vi "仁莫密封检测系统.vi"() -> ()   [LabVIEW 2015]
uses:
  <vilib>/NI/Modbus Library/API/Master/Modbus Master.lvclass
  <vilib>/Utility/file.llb/Read Delimited Spreadsheet (string).vi
  <vilib>/NI/Modbus Library/Transmission Data Unit/RTU/RTU Data Unit.lvclass
  <vilib>/NI/Modbus Library/Master Function Definition/Master Function Definition.lvclass
  <vilib>/NI/Modbus Library/Network Protocol/Network Master/Serial/Serial Master.lvclass
panel:
  out "扫码数据":string
  out "通讯状态":bool
  out "刷新按钮":bool
  out "参数组别":string
  out "测试时间":string
  out "实时压力":string
  out "泄露压力":string
  out "门限压力":string
  out "目标压力":string
  out "测试 NG":string
  out "测试 OK":string
  out "测试结果":string
  out "测试总量":string
  out "实时压力(图)":dbl(graph)
  in  "清除计数":bool
  in  "设备启动":bool
  out "消息框":string
  in  "设备停止":bool
  in  "阻断通讯":bool=TRUE
  out "运行状态":string
  out "失败原因":string
  in  "Exit":bool
  # "仁 莫 密 封 检 测 系 统"
  # "S"
  # "Pa"
  # "Pa"
  # "Pa"
  # "Pa"
  # "pcs"
  # "pcs"
  # "pcs"
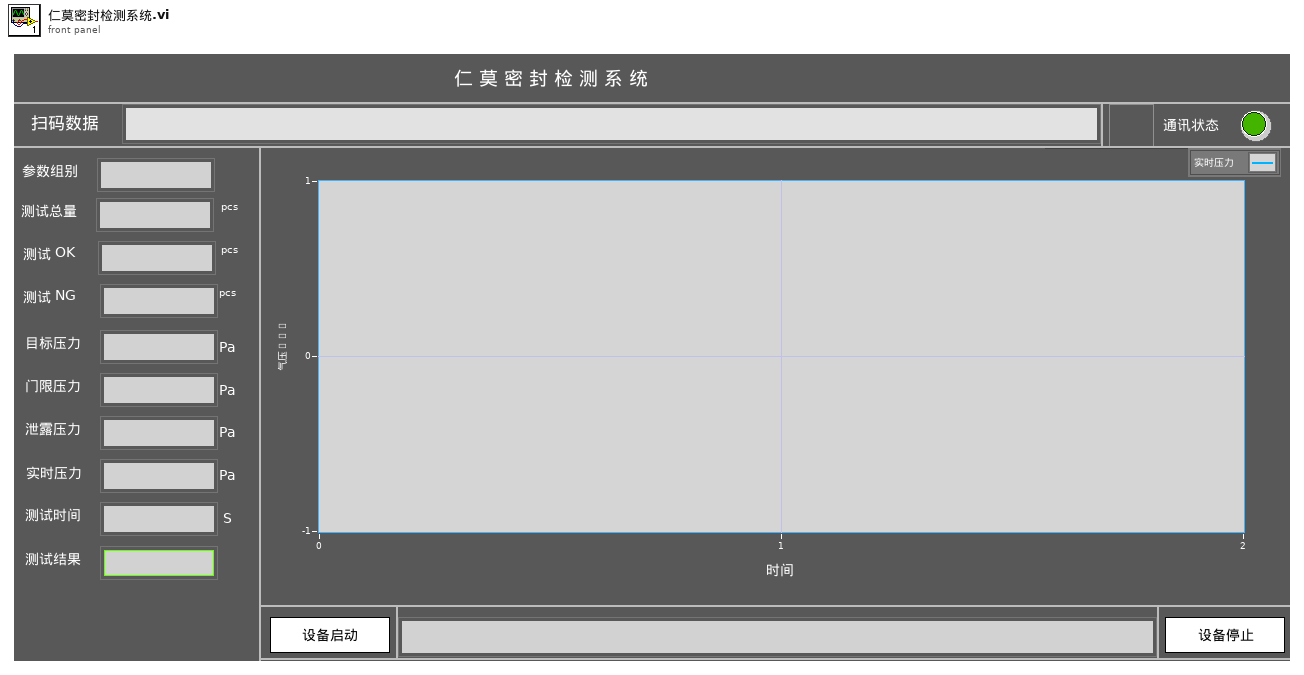
[diagram p1: front panel]
types:
  T1 = cluster{"地址":u16, "数量":u16, "寄存器值":u16[], "产品总数":string}[]
  T2 = enum32{"Invalid", "Standard", "Closed", "Hidden", "Minimized", "Maximized"}
  T3 = enum32{"invalid app kind", "Development System", "Run Time System", "Student Edition", "Embedded LabVIEW", "Evaluation", "Custom"}
  T4 = cluster{"地址":u16, "数量":u16, "寄存器值":u16[], "名称":string}[]
  T5 = cluster{"Core":cluster{"Current VI Reference":refnum<vi>, "Close Panel on Exit?":bool}, "serial master instance":refnum<class "Modbus Master.lvclass">, "进站OK":bool, "连接成功":bool, "正在运行":bool, "用户登录":bool, "A读保持寄存器信息组":cluster{"地址":u16, "数量":u16, "寄存器值":u16[], "名称":string}[], "A写入线圈信息组":cluster{"地址":u16, "布尔":bool, "名称":string}[], "A读多组线圈信息组":cluster{"地址":u16, "数量":u16, "名称":string, "线圈组":bool[]}[]}
  T6 = cluster{"读取信息簇":cluster{"地址":u16, "数量":u16, "寄存器值":u16[], "名称":string}, "值解析":string}[]
  T7 = cluster{"连接成功":bool, "MB_实体":refnum<class "Modbus Master.lvclass">}
  T8 = cluster{"地址":u16, "数量":u16, "名称":string, "线圈组":bool[]}[]
  T9 = cluster{"Current VI Reference":refnum<vi>, "Close Panel on Exit?":bool}
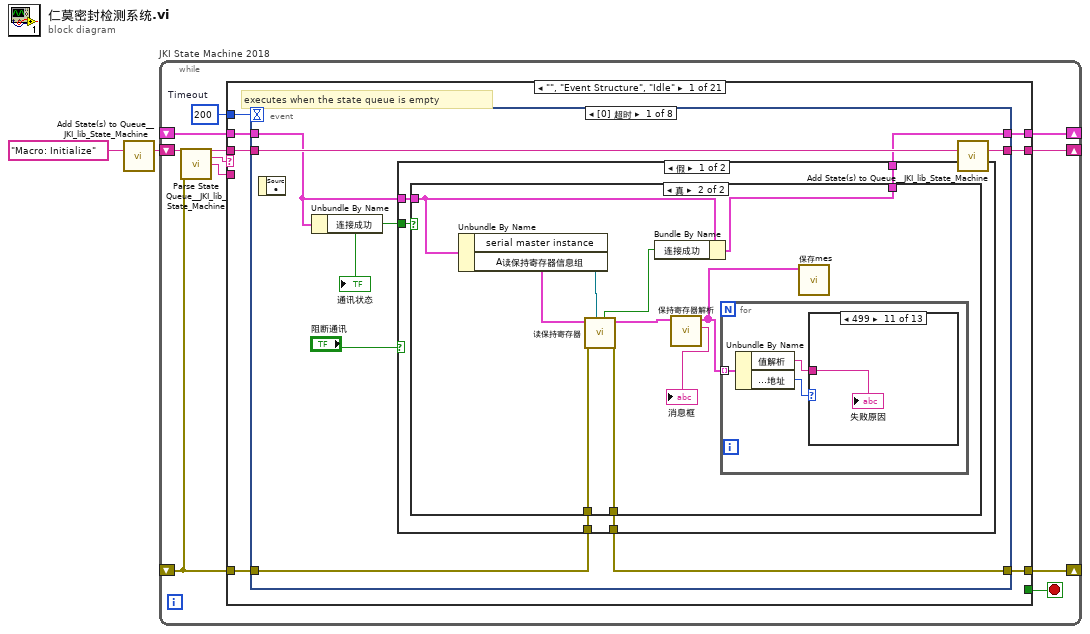
[diagram p0: block diagram]
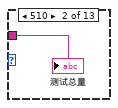
[diagram p4: hidden frame]
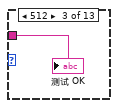
[diagram p5: hidden frame]
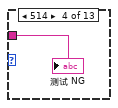
[diagram p6: hidden frame]
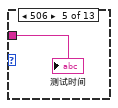
[diagram p7: hidden frame]
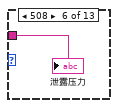
[diagram p8: hidden frame]
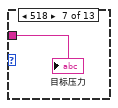
[diagram p9: hidden frame]
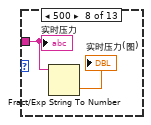
[diagram p10: hidden frame]
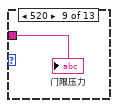
[diagram p11: hidden frame]
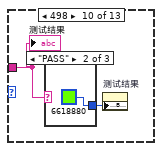
[diagram p12: hidden frame]
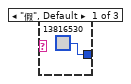
[diagram p13: hidden frame]
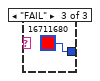
[diagram p14: hidden frame]
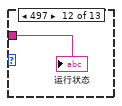
[diagram p15: hidden frame]
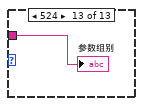
[diagram p16: hidden frame]
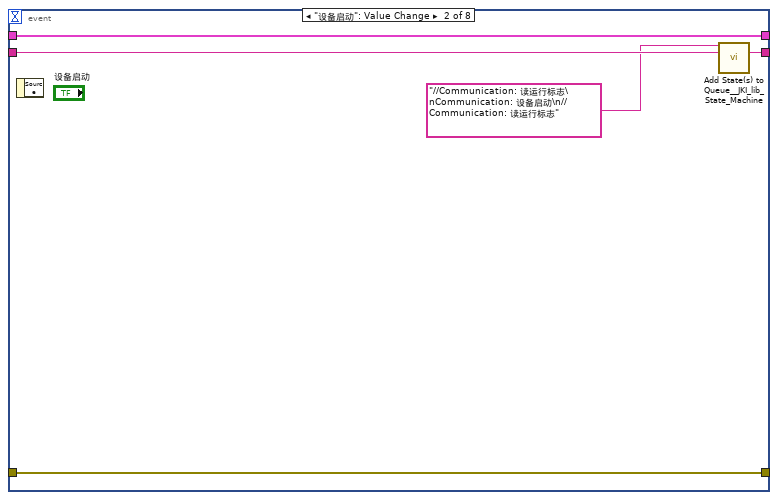
[diagram p18: hidden frame]
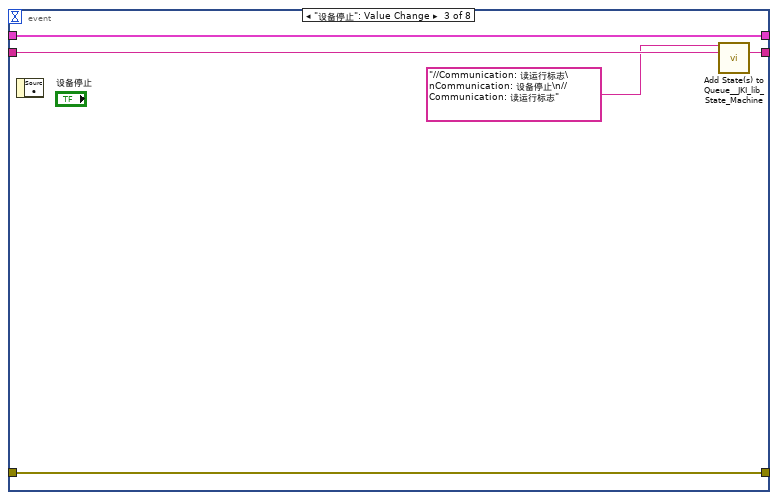
[diagram p19: hidden frame]
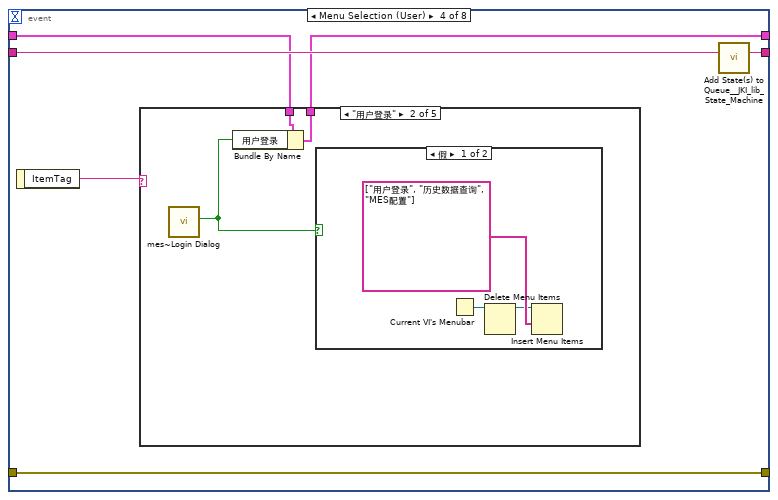
[diagram p20: hidden frame]
diagram:
  n1 = call <vilib>:"Add State(s) to Queue__JKI_lib_State_Machine.vi"("State(s) in (\"\")"="Macro: Initialize") -> ("States Out"=w2:string)  [unwired: 14 in]
  n2 = while "JKI State Machine 2018" {
    shift-right: [w6] -> _
    shift-left: _ -> [w5]
    shift-right: [w9] -> _
    shift-left: _ -> [w3]
    shift-right: [w8] -> _
    shift-left: w2 -> [w10]
    stop <- w7 stop-if-true
    w4 = 200  # Timeout
    n3 = call <vilib>:"Parse State Queue__JKI_lib_State_Machine.vi"("State Queue"=w10, "Error In (no error)"=w3) -> ("Remaining States"=w12:string, "Current State"=w13:string, "Arguments"=w11:string)  [unwired: 11 in]
    n4 = case shown="\"\", \"Event Structure\", \"Idle\"" w13 {
      selector: w13 -> [_ _ w156 _ _ _ _ _ _ _ _ _ _ _ _ _ _ _ _ _ _]
      tunnel: w12 -> [w20 w155 w160 w179 w186 w191 w195 w214 w222 w226 w240 w246 w257 w326 w331 w341 w345 w356 w370 w419 w462]
      tunnel: w11 -> [_ _ _ _ _ _ _ _ _ _ _ w241 w251 _ _ _ _ _ _ _ _]
      tunnel: w5 -> [w18 w152 w158 w172 w183 w189 w192 _ w218 w223 w238 w244 w253 w323 w328 w338 w342 w349 w364 w413 w455]
      tunnel: [w17 w153 w162 w176 errorcluster {"status"=FALSE, "code"=0, "source"=""} ("error out") w188 w193 w211 w219 w224 w237 w242 w254 w324 w329 w339 w343 w350 w367 w416 w459] -> w9
      tunnel: w3 -> [w16 w153 w161 w176 w181 w188 w193 w211 w216 w224 w237 w243 w255 w324 w329 w339 w343 w353 w368 w417 w460]
      tunnel: [w19 w154 w159 w178 w185 w190 w194 w213 w221 w225 w239 w245 w256 w325 w330 w340 w344 w355 w369 w418 w461] -> w8
      tunnel: [_ _ _ _ _ TRUE _ _ _ _ _ _ _ _ _ _ _ _ _ _ _] -> w7
      tunnel: [w15 w152 w158 w177 w183 w189 w192 w212 w218 w223 w238 w244 w253 w323 w328 w338 w342 w347 w362 w411 w456] -> w6
      tunnel: w4 -> [w14 _ _ _ _ _ _ _ _ _ _ _ _ _ _ _ _ _ _ _ _]
      frame "", "Event Structure", "Idle" {
        # "executes when the state queue is empty"
        n5 = event shown="[0] 超时" {
          selector: _ -> [_ _ _ _ _ _ _ _]
          dyn-events: _ -> [_ _ _ _ _ _ _ _]
          timeout: w14 -> [_ _ _ _ _ _ _ _]
          tunnel: w20 -> [w28 w72 w77 w83 w124 w135 w145 w151]
          tunnel: [w27 w71 w76 w82 w123 w134 w144 w150] -> w19
          tunnel: w18 -> [w26 w69 w74 w79 w119 w130 w142 w148]
          tunnel: [w24 w70 w75 w81 w122 w127 w143 w149] -> w17
          tunnel: w16 -> [w25 w70 w75 w81 w122 w128 w143 w149]
          tunnel: [w23 w69 w74 w78 w117 w129 w142 w148] -> w15
          event Timeout {
            n6 = event-data() -> ()  [unwired: 1 in, 1 out]
            n7 = Unbundle By Name(w26) -> ("连接成功"=w21:bool)
            "通讯状态" <- w21
            n8 = case shown="假" "阻断通讯" {
              tunnel: w21 -> [w33 _]
              tunnel: w26 -> [w32 w66]
              tunnel: w25 -> [w31 w67]
              tunnel: [w30 w67] -> w24
              tunnel: [w29 w66] -> w23
              frame False {
                n9 = case shown="真" w33 {
                  tunnel: w32 -> [w35 w43]
                  tunnel: w31 -> [w34 w45]
                  tunnel: [w34 w44] -> w30
                  tunnel: [w35 w37] -> w29
                  frame False {
                  }
                  frame True {
                    n10 = Unbundle By Name(w43) -> ("serial master instance"=w42:refnum<class "Modbus Master.lvclass">, "A读保持寄存器信息组"=w41:T4)
                    n11 = call "读保持寄存器.vi"("MB_实体"=w42, "error in"=w45, "读保持寄存器信息组__输入"=w41) -> ("输出簇"=w44:errorcluster, "读保持寄存器信息组_输出"=w39:T4, "连接成功"=w40:bool)  [unwired: 6 in]
                    n12 = Bundle By Name(cluster=w43, "连接成功"=w40) -> (w37:T5)
                    n13 = call "保持寄存器解析.vi"("A读保持寄存器信息组"=w39) -> ("运行状态"=→"消息框":string, "参数值"=w36:T6)  [unwired: 9 in]
                    n14 = for {
                      tunnel: w36 -> [w47] mode=indexing
                      n15 = Unbundle By Name(w47) -> ("值解析"=w46:string, "读取信息簇.地址"=w48:u16)
                      n16 = case shown="499" w48 {
                        tunnel: w46 -> [_ w49 w50 w51 w52 w53 w54 w56 w57 w59 w63 w64 w65]
                        frame Default {
                        }
                        frame 510 {
                          "测试总量" <- w49
                        }
                        frame 512 {
                          "测试 OK" <- w50
                        }
                        frame 514 {
                          "测试 NG" <- w51
                        }
                        frame 506 {
                          "测试时间" <- w52
                        }
                        frame 508 {
                          "泄露压力" <- w53
                        }
                        frame 518 {
                          "目标压力" <- w54
                        }
                        frame 500 {
                          n17 = Fract/Exp String To Number(string=w56) -> (number=→"实时压力(图)":dbl)  [unwired: 3 in, 1 out]
                          "实时压力" <- w56
                        }
                        frame 520 {
                          "门限压力" <- w57
                        }
                        frame 498 {
                          n18 = case shown="\"PASS\"" w59 {
                            tunnel: [u32 13816530 ("颜色盒") u32 6618880 u32 16711680] -> w58
                            frame "假", Default {
                            }
                            frame "PASS" {
                            }
                            frame "FAIL" {
                            }
                          }
                          n19 = property on="测试结果" class="Str"("Text.BGColor"=w58) -> ()  [unwired: 2 in, 2 out]
                          "测试结果" <- w59
                        }
                        frame 499 {
                          "失败原因" <- w63
                        }
                        frame 497 {
                          "运行状态" <- w64
                        }
                        frame 524 {
                          "参数组别" <- w65
                        }
                      }
                    }
                    n20 = call "保存mes.vi"("参数值"=w36) -> ()  [unwired: 11 in]
                  }
                }
              }
              frame True {
              }
            }
            n21 = call <vilib>:"Add State(s) to Queue__JKI_lib_State_Machine.vi"("State(s) in (\"\")"=w28) -> ("States Out"=w27:string)  [unwired: 14 in]
          }
          event "设备启动": Value Change {
            n22 = event-data() -> ()  [unwired: 1 in, 1 out]
            n23 = call <vilib>:"Add State(s) to Queue__JKI_lib_State_Machine.vi"("State(s) in Front (\"\")"="//Communication: 读运行标志\nCommunication: 设备启动\n//Communication: 读运行标志", "State(s) in (\"\")"=w72) -> ("States Out"=w71:string)  [unwired: 13 in]
          }
          event "设备停止": Value Change {
            n24 = event-data() -> ()  [unwired: 1 in, 1 out]
            n25 = call <vilib>:"Add State(s) to Queue__JKI_lib_State_Machine.vi"("State(s) in Front (\"\")"="//Communication: 读运行标志\nCommunication: 设备停止\n//Communication: 读运行标志", "State(s) in (\"\")"=w77) -> ("States Out"=w76:string)  [unwired: 13 in]
          }
          event Menu Selection (User) {
            n26 = event-data() -> ("ItemTag"=w80:string)  [unwired: 1 in]
            n27 = case shown="\"用户登录\"" w80 {
              tunnel: w79 -> [w84 w87 w95 w106 w108]
              tunnel: [w84 w86 w95 w106 w107] -> w78
              frame "假", Default {
              }
              frame "用户登录" {
                n28 = call "mes~Login Dialog.vi"() -> ("Success?"=w85:bool)  [unwired: 11 in]
                n29 = Bundle By Name(cluster=w87, "用户登录"=w85) -> (w86:T5)
                n30 = case shown="假" w85 {
                  frame False {
                    n31 = Current VI's Menubar() -> (w89:refnum<k9>)
                    n32 = Delete Menu Items(9:w89) -> (3:w88:refnum<k9>)  [unwired: 3 in, 1 out]
                    n33 = Insert Menu Items(7:string[] ["用户登录", "历史数据查询", "MES配置"] ("L10n_item tags 1"), 9:w88) -> ()  [unwired: 4 in, 3 out]
                  }
                  frame True {
                    n34 = Current VI's Menubar() -> (w93:refnum<k9>)
                    n35 = Delete Menu Items(9:w93) -> (0:w91:errorcluster, 3:w92:refnum<k9>)  [unwired: 3 in]
                    n36 = Insert Menu Items(6:w91, 7:string[] ["用户登录", "历史数据查询", "通讯参数设置", "MES配置"] ("L10n_item tags 1"), 9:w92) -> ()  [unwired: 3 in, 3 out]
                  }
                }
              }
              frame "历史数据查询" {
                n37 = stacked-sequence {
                  frame #0 {
                    n38 = call <vilib>:"Check if File or Folder Exists.vi"("path"=path "D:/MES" ("路径")) -> ("file or folder exists?"=w98:bool, "dup path"=w97:path)  [unwired: 8 in, 1 out]
                    n39 = case shown="假" w98 {
                      tunnel: w97 -> [w100 w101]
                      tunnel: [w99 w101] -> _
                      frame False {
                        n40 = Create Folder(path (use dialog)=w100) -> (created path=w99:path)  [unwired: 2 in, 2 out]
                      }
                      frame True {
                      }
                    }
                  }
                  frame #1 {
                    n41 = call <vilib>:"Space Constant.vi"() -> ("String"=w103:string)
                    n42 = Concatenate Strings("explorer" ("字符串"), w103, "D:\\MES" ("字符串")) -> (w105:string)
                    n43 = call <vilib>:"System Exec.vi"("command line"=w105) -> ()  [unwired: 7 in, 4 out]
                  }
                }
              }
              frame "MES配置" {
                n44 = call "mes参数配置.vi"() -> ()  [unwired: 12 in]
              }
              frame "通讯参数设置" {
                n45 = stacked-sequence {
                  tunnel: w108 -> [_ w113 _]
                  tunnel: [_ w110 _] -> w107
                  frame #0 {
                    n46 = local write "阻断通讯"(TRUE ("阻断通讯")) -> ()
                  }
                  frame #1 {
                    n47 = call "通讯参数设置.vi"() -> ("A设备簇"=w114:T7)  [unwired: 5 in]
                    n48 = Unbundle By Name(w114) -> ("MB_实体"=w112:refnum<class "Modbus Master.lvclass">, "连接成功"=w111:bool)
                    n49 = Bundle By Name(cluster=w113, "serial master instance"=w112, "连接成功"=w111) -> (w110:T5)
                  }
                  frame #2 {
                    n50 = local write "阻断通讯"(FALSE ("阻断通讯")) -> ()
                  }
                }
              }
            }
            n51 = call <vilib>:"Add State(s) to Queue__JKI_lib_State_Machine.vi"("State(s) in (\"\")"=w83) -> ("States Out"=w82:string)  [unwired: 14 in]
          }
          event "扫码数据", "刷新按钮": Mouse Down {
            n52 = event-data() -> ()  [unwired: 1 in, 1 out]
            n53 = call "扫码页面.vi"() -> ("Return"=w120:string)  [unwired: 3 in]
            "扫码数据" <- w120
            n54 = global write "Global.vi" "PACK编码"(w120) -> ()
            n55 = call "mes~产品进站.vi"("identification"=w120) -> ("进站成功"=w118:bool)  [unwired: 9 in, 1 out]
            n56 = case shown="真" w118 {
              tunnel: ["产品进站失败，请重新扫码。" "产品进站成功。"] -> w116
              frame False {
              }
              frame True {
              }
            }
            n57 = Bundle By Name(cluster=w119, "进站OK"=w118) -> (w117:T5)
            n58 = local write "消息框"(w116) -> ()
            n59 = call <vilib>:"Add State(s) to Queue__JKI_lib_State_Machine.vi"("State(s) in (\"\")"=w124) -> ("States Out"=w123:string)  [unwired: 14 in]
            "刷新按钮" <- FALSE ("刷新按钮")
          }
          event "清除计数": Value Change {
            n60 = event-data() -> ()  [unwired: 1 in, 1 out]
            n61 = local write "清除计数"(FALSE) -> ()
            n62 = Unbundle By Name(w130) -> ("serial master instance"=w131:refnum<class "Modbus Master.lvclass">)
            n63 = disable-structure shown="禁用" {
              disable-tunnel: [w140 _] -> w132
              disable-tunnel: w131 -> [w139 _]
              disable-tunnel: w128 -> [w137 _]
              disable-tunnel: [w136 _] -> w127
              frame Disabled {
                n64 = call "写保持寄存器.vi"("MB_实体"=w139, "error in"=w137, "读保持寄存器信息组__输入"=T1 [{"地址"=510, "数量"=2, "寄存器值"=[0, 0], "产品总数"="产品总数"}, {"地址"=512, "数量"=2, "寄存器值"=[0, 0], "产品总数"="合格数量"}, {"地址"=514, "数量"=2, "寄存器值"=[0, 0], "产品总数"="泄露数量"}]) -> ("输出簇"=w136:errorcluster, "连接成功"=w140:bool)  [unwired: 7 in]
              }
              frame Enabled {
              }
            }
            n65 = Bundle By Name(cluster=w130, "连接成功"=w132) -> (w129:T5)
            n66 = call <vilib>:"Add State(s) to Queue__JKI_lib_State_Machine.vi"("State(s) in (\"\")"=w135) -> ("States Out"=w134:string)  [unwired: 14 in]
          }
          event "Exit": Value Change {
            # "Exit Button Value Change (pressed) Event\n(this executes Macro: Exit to terminate the VI)"
            n67 = event-data() -> ()  [unwired: 1 in, 1 out]
            n68 = call <vilib>:"Add State(s) to Queue__JKI_lib_State_Machine.vi"("State(s) in Front (\"\")"="Macro: Exit", "State(s) in (\"\")"=w145) -> ("States Out"=w144:string)  [unwired: 13 in]
          }
          event Panel Close? {
            # "Discard the event because we'll close the front panel ourselves in Macro: Exit"
            # "Close Panel button (pressed) Event\n(this executes Macro: Exit to terminate the VI)"
            n69 = event-data() -> ()  [unwired: 1 in, 1 out]
            n70 = event-data("Discard?"=TRUE) -> ()  [unwired: 1 in, 1 out]
            n71 = call <vilib>:"Add State(s) to Queue__JKI_lib_State_Machine.vi"("State(s) in Front (\"\")"="Macro: Exit", "State(s) in (\"\")"=w151) -> ("States Out"=w150:string)  [unwired: 13 in]
          }
        }
      }
      frame "---------- Core ----------" {
        # "Do not put any code in this frame.\n(it is a separator no-op)"
        n72 = call <vilib>:"Add State(s) to Queue__JKI_lib_State_Machine.vi"("State(s) in (\"\")"=w155) -> ("States Out"=w154:string)  [unwired: 14 in]
      }
      frame Default {
        w165 = 42 items=["No error", "Argument error", "Memory is full", "Out of zone", "End of file", "File already open", "Generic file I/O error", "File not found", "File permission error", "Disk is full", "Duplicate path", "Too many files open", "System feature not enabled", "Resource file not found", "Cannot add resource", "Resource not found", "Image not found", "Image memory error", "Pen does not exist", "Config type invalid", "Config token not found", "Config parse error", "Config memory error", "Bad external code format", "Bad external code offset", "External code not present", "Null window", "Destroy window error", "Null menu", "Print aborted", "Bad print record", "Print driver error", "Windows error during printing", "Memory error during printing", "Print dialog error", "Generic print error", "Invalid device refnum", "Device not found", "Device parameter error", "Device unit error", "Cannot open device", "Device call aborted", "Generic error", "Cancelled by user", "Object ID too low", "Object ID too high", "Object not in heap", "Unknown heap", "Unknown object (invalid DefProc)", "Unknown object (DefProc not in table)", "Message out of range", "Invalid (null) method", "Unknown message", "Manager call not supported", "Bad address", "Network operation in progress", "Network operation timed out", "Connection is busy", "Network attribute not supported", "Network error", "Address in use", "System out of memory", "Connection aborted", "Connection refused", "Not connected", "Already connected", "Connection closed", "Initialization error (interapplication manager)", "Bad occurrence", "Wait on unbound occurrence handler", "Occurrence queue overflow", "Datalog type conflict", "Unused", "Unrecognized type (interapplication manager)", "Memory corrupt", "Failed to make temporary DLL", "Old CIN version", "Drag socket not found", "Failed to load drop-object", "Failed to register OLE object", "Failed to release OLE object", "Format specifier type mismatch", "Unknown format specifier", "Too few format specifiers", "Too many format specifiers", "Scan failed", "Newer CIN version", "Error converting to variant", "Runtime menu error", "Password tampered", "Variant attribute not found", "Incompatible variant data type", "Event data is not available", "Event Store is not present", "Occurrence is not found", "Event Queue is not created", "Event info is not available", "Refnum passed is NULL", "Error retrieving Class GUID", "Error retrieving CoClass GUID", "Error retrieving TypeLib GUID.", "Bad built application magic bytes.", "Specific driver is different from the specific driver associated with the Logical Name.", "There is no session opened to the class driver.", "Max Error", "MAX - Error with config objects", "MAX - Error loading configuration", "MAX - Group not supported"]
        # "Current State"
        # "Do not delete, rename, or modify this frame.\n(this is used to capture unhandled states and typos)"
        # "Handle mistyped state name (developer tool)"
        n73 = Format Into String(format string="Software Exception: Unhandled State \"%s\"." ("message"), error in=w161, w156) -> (resulting string=w164:string, error out=w163:errorcluster)  [unwired: 1 in]
        n74 = call <vilib>:"Error Cluster From Error Code.vi"("show call chain? (False)"=TRUE, "error in (no error)"=w163, "error message (\"\")"=w164, "error code (0)"=w165) -> ("error out"=w162:errorcluster)  [unwired: 5 in]
        n75 = call <vilib>:"Add State(s) to Queue__JKI_lib_State_Machine.vi"("State(s) in (\"\")"=w160) -> ("States Out"=w159:string)  [unwired: 14 in]
      }
      frame "Initialize Core Data" {
        # "Do not delete, rename, or modify this frame.\n(this is used to determine panel behavior on exit)"
        # "originally closed?"
        # "exe?"
        # "If panel starts closed or is an EXE, then close it when we exit"
        n76 = property class="VI"() -> ("FP.State"=w169:T2)  [unwired: 2 in, 2 out]
        n77 = property class="App"() -> ("App.Kind"=w175:T3)  [unwired: 2 in, 2 out]
        n78 = control-ref of="Current VI Reference"() -> (w170:refnum<vi>)
        n79 = Equal?(x=w169, y=T2."Closed" ("Front Panel Window:State")) -> (x = y?=w167:bool)
        n80 = Equal?(x=w175, y=T3."Run Time System" ("Application:Kind")) -> (x = y?=w173:bool)
        n81 = Or(x=w167, y=w173) -> (x .or. y?=w171:bool)
        n82 = Bundle By Name(cluster=w172, "Core.Current VI Reference"=w170, "Core.Close Panel on Exit?"=w171) -> (w177:T5)
        n83 = call <vilib>:"Add State(s) to Queue__JKI_lib_State_Machine.vi"("State(s) in (\"\")"=w179) -> ("States Out"=w178:string)  [unwired: 14 in]
      }
      frame "Error Handler" {
        # "Handle any errors here.\nYou can also output any states to clean-up after errors occur"
        # "Clear error"
        n84 = Unbundle By Name(w181) -> ("source"=w180:string)
        n85 = One Button Dialog(message=w180) -> ()  [unwired: 1 in, 1 out]
        n86 = call <vilib>:"Add State(s) to Queue__JKI_lib_State_Machine.vi"("State(s) in Front (\"\")"="/* Post Error States", "State(s) in (\"\")"=w186) -> ("States Out"=w185:string)  [unwired: 13 in]
      }
      frame "Exit" {
        # "Do not put any code in this frame.\n(No errors that occur here will be handled.)"
        n87 = call <vilib>:"Add State(s) to Queue__JKI_lib_State_Machine.vi"("State(s) in (\"\")"=w191) -> ("States Out"=w190:string)  [unwired: 14 in]
      }
      frame "---------- Data ----------" {
        # "Do not put any code in this frame.\n(It is a separator no-op. You can make a copy of this frame to create a new Data frame)"
        n88 = call <vilib>:"Add State(s) to Queue__JKI_lib_State_Machine.vi"("State(s) in (\"\")"=w195) -> ("States Out"=w194:string)  [unwired: 14 in]
      }
      frame "Data: Initialize" {
        w196 = FALSE  # 进站OK
        w203 = FALSE  # 用户登录
        w204 = FALSE  # 正在运行
        w205 = T4 [{"地址"=510, "数量"=2, "寄存器值"=[0, 0], "名称"="产品总数"}, {"地址"=512, "数量"=2, "寄存器值"=[0, 0], "名称"="合格数量"}, {"地址"=514, "数量"=2, "寄存器值"=[0, 0], "名称"="泄露数量"}, {"地址"=506, "数量"=2, "寄存器值"=[0, 0], "名称"="1测试时间"}, {"地址"=508, "数量"=2, "寄存器值"=[0, 0], "名称"="1测试泄漏"}, {"地址"=518, "数量"=2, "寄存器值"=[0, 0], "名称"="1#目标压力"}, {"地址"=498, "数量"=1, "寄存器值"=[0, 0], "名称"="1#测试结果"}, {"地址"=500, "数量"=2, "寄存器值"=[0, 0], "名称"="实时压力"}, {"地址"=520, "数量"=2, "寄存器值"=[], "名称"="门限压力"}, {"地址"=499, "数量"=1, "寄存器值"=[], "名称"="失败原因"}, {"地址"=497, "数量"=1, "寄存器值"=[], "名称"="运行状态"}, {"地址"=524, "数量"=2, "寄存器值"=[], "名称"="参数组别"}]  # A读保持寄存器信息组
        w206 = T8 [{"地址"=507, "数量"=1, "名称"="1测试结束标志", "线圈组"=[FALSE, TRUE]}]  # A读多组线圈信息组
        w207 = cluster{"地址":u16, "布尔":bool, "名称":string}[] [{"地址"=50, "布尔"=FALSE, "名称"="启动"}, {"地址"=51, "布尔"=FALSE, "名称"="停止"}]  # A写入线圈信息组
        w208 = FALSE  # 连接成功
        w209 = refnum<class "Modbus Master.lvclass"> refnum  # serial master instance
        w210 = T9 {"Current VI Reference"=refnum, "Close Panel on Exit?"=FALSE}  # Core
        # "Data names and types of shift register data are defined by this bundle."
        # "Initialize the shift-register data, here.\n(data names are defined by what you wire into the bundle function)"
        n89 = call <vilib>:"Application Directory.vi"() -> ("Application Directory"=w201:path)
        n90 = Build Path(base path=w201, name or relative path=path "data/mes.cfg") -> (appended path=w202:path)
        n91 = call-poly <vilib>:"Read Delimited Spreadsheet.vi"("file path (dialog if empty)"=w202, "delimiter (\\t)"="::" ("delimiter (\\t)")) -> ("all rows"=w197:string[][])  [unwired: 8 in, 5 out]
        n92 = call "mes初始化.vi"("mes"=w197) -> ()  [unwired: 11 in]
        n93 = global write "Global.vi" "运行状态时间点"(dbl[] [0.0, 0.0, 0.0, 0.0, 0.0, 0.0, 0.0, 0.0, 0.0] ("运行状态时间点")) -> ()
        n94 = Bundle("Core"=w210, "serial master instance"=w209, "进站OK"=w196, "连接成功"=w208, "正在运行"=w204, "用户登录"=w203, "A读保持寄存器信息组"=w205, "A写入线圈信息组"=w207, "A读多组线圈信息组"=w206) -> (w212:T5)  [unwired: 1 in]
        n95 = call <vilib>:"Add State(s) to Queue__JKI_lib_State_Machine.vi"("State(s) in (\"\")"=w214) -> ("States Out"=w213:string)  [unwired: 14 in]
      }
      frame "Data: Cleanup" {
        # "Cleanup any data and references, here.\n(this is called automatically, by the Macro: Exit)"
        n96 = Unbundle By Name(w218) -> ("Core.Current VI Reference"=w220:refnum<vi>, "serial master instance"=w217:refnum<class "Modbus Master.lvclass">)
        n97 = call-dynamic "Shutdown.vi"("error in"=w216, "Modbus master in"=w217) -> ("error out"=w215:errorcluster)  [unwired: 9 in]
        n98 = Close Reference(reference=w220, error in (no error)=w215) -> (error out=w219:errorcluster)
        n99 = call <vilib>:"Add State(s) to Queue__JKI_lib_State_Machine.vi"("State(s) in (\"\")"=w222) -> ("States Out"=w221:string)  [unwired: 14 in]
      }
      frame "---------- UI ----------" {
        # "Do not put any code in this frame.\n(It is a separator no-op. You can make a copy of this frame to create a new UI frame)"
        n100 = call <vilib>:"Add State(s) to Queue__JKI_lib_State_Machine.vi"("State(s) in (\"\")"=w226) -> ("States Out"=w225:string)  [unwired: 14 in]
      }
      frame "UI: Initialize" {
        w232 = ""
        # "Initialize the User Interface, here.\n(this is called automatically, by the Macro: Init)"
        n101 = call "读取配置文件.vi"("配置"="程序名") -> ("error out"=w231:errorcluster, "路径"=w230:string)  [unwired: 9 in]
        n102 = property class="VI"(error in=w231, "Front Panel.Title"=w230) -> (error out=w228:errorcluster)  [unwired: 1 in, 1 out]
        n103 = Current VI's Menubar() -> (w236:refnum<k9>)
        n104 = Delete Menu Items(6:w228, 9:w236) -> (0:w235:errorcluster, 3:w234:refnum<k9>)  [unwired: 2 in]
        n105 = local write "扫码数据"(w232) -> ()
        n106 = global write "Global.vi" "PACK编码"(w232) -> ()
        n107 = Insert Menu Items(6:w235, 7:string[] ["用户登录", "历史数据查询", "MES配置"] ("L10n_item tags 1"), 9:w234) -> ()  [unwired: 3 in, 3 out]
        n108 = property on="测试结果" class="Str"("Text.BGColor"=u32 13816530 ("颜色盒")) -> ()  [unwired: 2 in, 2 out]
        n109 = call <vilib>:"Add State(s) to Queue__JKI_lib_State_Machine.vi"("State(s) in (\"\")"=w240) -> ("States Out"=w239:string)  [unwired: 14 in]
      }
      frame "UI: Cursor Set" {
        # "Argument"
        # "Set and Unset Cursor Busy.\n(Usage: \"UI: Cursor Set >> Busy|Idle\")"
        n110 = case shown="\"Idle\", 默认" w241 {
          tunnel: w243 -> [w248 w250]
          tunnel: [w247 w249] -> w242
          frame "Idle", Default {
            n111 = call <vilib>:"Unset Busy.vi"("error in (no error)"=w248) -> ("error out"=w247:errorcluster)  [unwired: 10 in]
          }
          frame "Busy" {
            n112 = call <vilib>:"Set Busy.vi"("error in (no error)"=w250) -> ("error out"=w249:errorcluster)  [unwired: 9 in, 1 out]
          }
        }
        n113 = call <vilib>:"Add State(s) to Queue__JKI_lib_State_Machine.vi"("State(s) in (\"\")"=w246) -> ("States Out"=w245:string)  [unwired: 14 in]
      }
      frame "UI: Front Panel State" {
        # "Argument"
        # "Set Front Panel Open or Closed\n(Usage: \"UI: Front Panel State >> Open|Close\")"
        n114 = Unbundle By Name(w253) -> ("Core.Current VI Reference"=w252:refnum<vi>)
        n115 = case shown="\"Maximize\", \"Maximized\"" w251 {
          tunnel: w255 -> [w263 w278 w289 w302 w315]
          tunnel: [w265 w279 w291 w304 w317] -> w254
          tunnel: w252 -> [w264 w276 w290 w303 w316]
          frame "Open", "Standard", Default {
            w258 = T2."Standard" ("State")
            n116 = property class="VI"(reference=w264, error in=w263) -> (reference out=w261:refnum<vi>, error out=w262:errorcluster, "FP.State"=w260:T2)
            n117 = Not Equal?(x=w260, y=w258) -> (x != y?=w259:bool)
            n118 = case shown="真" w259 {
              tunnel: [w269 w271] -> w265
              tunnel: w262 -> [w268 w271]
              tunnel: w261 -> [w267 _]
              tunnel: w258 -> [w266 _]
              frame True {
                n119 = invoke class="VI" method="FP.Open"(reference=w267, error in=w268, "Activate"=TRUE, "State"=w266) -> (error out=w269:errorcluster)  [unwired: 1 in, 4 out]
              }
              frame False {
              }
            }
          }
          frame "Close", "Closed" {
            n120 = property class="VI"(reference=w276, error in=w278) -> (reference out=w275:refnum<vi>, error out=w277:errorcluster, "FP.State"=w273:T2)
            n121 = Not Equal?(x=w273, y=T2."Closed" ("Front Panel Window:State")) -> (x != y?=w272:bool)
            n122 = case shown="真" w272 {
              tunnel: [w280 w283] -> w279
              tunnel: w277 -> [w280 w282]
              tunnel: w275 -> [_ w281]
              frame False {
              }
              frame True {
                n123 = invoke class="VI" method="FP.Close"(reference=w281, error in=w282) -> (error out=w283:errorcluster)  [unwired: 1 in, 2 out]
              }
            }
          }
          frame "Hidden", "Hide" {
            w284 = T2."Hidden" ("State")
            n124 = property class="VI"(reference=w290, error in=w289) -> (reference out=w287:refnum<vi>, error out=w288:errorcluster, "FP.State"=w286:T2)
            n125 = Not Equal?(x=w286, y=w284) -> (x != y?=w285:bool)
            n126 = case shown="真" w285 {
              tunnel: [w295 w296] -> w291
              tunnel: w288 -> [w294 w296]
              tunnel: w287 -> [w293 _]
              tunnel: w284 -> [w292 _]
              frame True {
                n127 = invoke class="VI" method="FP.Open"(reference=w293, error in=w294, "State"=w292) -> (error out=w295:errorcluster)  [unwired: 2 in, 4 out]
              }
              frame False {
              }
            }
          }
          frame "Minimize", "Minimized" {
            w297 = T2."Minimized" ("State")
            n128 = property class="VI"(reference=w303, error in=w302) -> (reference out=w300:refnum<vi>, error out=w301:errorcluster, "FP.State"=w299:T2)
            n129 = Not Equal?(x=w299, y=w297) -> (x != y?=w298:bool)
            n130 = case shown="真" w298 {
              tunnel: [w308 w309] -> w304
              tunnel: w301 -> [w307 w309]
              tunnel: w300 -> [w306 _]
              tunnel: w297 -> [w305 _]
              frame True {
                n131 = invoke class="VI" method="FP.Open"(reference=w306, error in=w307, "State"=w305) -> (error out=w308:errorcluster)  [unwired: 2 in, 4 out]
              }
              frame False {
              }
            }
          }
          frame "Maximize", "Maximized" {
            w310 = T2."Maximized" ("State")
            n132 = property class="VI"(reference=w316, error in=w315) -> (reference out=w313:refnum<vi>, error out=w314:errorcluster, "FP.State"=w312:T2)
            n133 = Not Equal?(x=w312, y=w310) -> (x != y?=w311:bool)
            n134 = case shown="真" w311 {
              tunnel: [w321 w322] -> w317
              tunnel: w314 -> [w320 w322]
              tunnel: w313 -> [w319 _]
              tunnel: w310 -> [w318 _]
              frame True {
                n135 = invoke class="VI" method="FP.Open"(reference=w319, error in=w320, "State"=w318) -> (error out=w321:errorcluster)  [unwired: 2 in, 4 out]
              }
              frame False {
              }
            }
          }
        }
        n136 = call <vilib>:"Add State(s) to Queue__JKI_lib_State_Machine.vi"("State(s) in (\"\")"=w257) -> ("States Out"=w256:string)  [unwired: 14 in]
      }
      frame "---------- Macro ----------" {
        # "Do not put any code in this frame.\n(It is a separator no-op. You can make a copy of this frame to create a new Macro frame)"
        n137 = call <vilib>:"Add State(s) to Queue__JKI_lib_State_Machine.vi"("State(s) in (\"\")"=w326) -> ("States Out"=w325:string)  [unwired: 14 in]
      }
      frame "Macro: Initialize" {
        w327 = "Data: Initialize\nInitialize Core Data\nUI: Initialize\nUI: Front Panel State >> Maximize\nCommunication: Open Serial\nCommunication: 读运行标志"  # Data: Initialize Initialize Core Data UI: Initialize UI: Front Panel State >> Maximize Communication: Open Serial Communication: 读运行标志
        # "Initialization Macro\n(This is called once, when the VI starts)"
        n138 = call <vilib>:"Add State(s) to Queue__JKI_lib_State_Machine.vi"("State(s) in Front (\"\")"=w327, "State(s) in (\"\")"=w331) -> ("States Out"=w330:string)  [unwired: 13 in]
      }
      frame "Macro: Exit" {
        # "Exit Macro\n(This is called once, when the VI exits)"
        n139 = Unbundle By Name(w338) -> ("Core.Close Panel on Exit?"=w337:bool)
        n140 = Select(t="UI: Front Panel State >> Close", s=w337, f="") -> (s? t:f=w334:string)
        n141 = call <vilib>:"Add State(s) to Queue__JKI_lib_State_Machine.vi"("State(s) in (\"\")"=w334, "State(s) at Back (\"\")"="Data: Cleanup\nExit") -> ("States Out"=w332:string)  [unwired: 13 in]
        n142 = call <vilib>:"Add State(s) to Queue__JKI_lib_State_Machine.vi"("State(s) in Front (\"\")"=w332, "State(s) in (\"\")"=w341) -> ("States Out"=w340:string)  [unwired: 13 in]
      }
      frame "---------- Communication ----------" {
        # "Template Separator\n(You can make a copy of, or modify, this frame)"
        n143 = call <vilib>:"Add State(s) to Queue__JKI_lib_State_Machine.vi"("State(s) in (\"\")"=w345) -> ("States Out"=w344:string)  [unwired: 14 in]
      }
      frame "Communication: Open Serial" {
        # "Your code here.\n(You can make a copy of, or modify, this frame)"
        n144 = call "读取配置文件.vi"("error in"=w353, "配置"="串口号") -> ("error out"=w352:errorcluster, "路径"=w351:string)  [unwired: 8 in]
        n145 = call "开机连接.vi"("error in"=w352, "串口号"=w351) -> ("error out"=w350:errorcluster, "连接成功"=w346:bool, "serial master instance"=w348:refnum<class "Modbus Master.lvclass">)  [unwired: 7 in]
        n146 = Bundle By Name(cluster=w349, "serial master instance"=w348, "连接成功"=w346) -> (w347:T5)
        n147 = call <vilib>:"Add State(s) to Queue__JKI_lib_State_Machine.vi"("State(s) in (\"\")"=w356) -> ("States Out"=w355:string)  [unwired: 14 in]
      }
      frame "Communication: 设备启动" {
        # "Your code here.\n(You can make a copy of, or modify, this frame)"
        n148 = Unbundle By Name(w364) -> ("serial master instance"=w365:refnum<class "Modbus Master.lvclass">, "连接成功"=w366:bool, "用户登录"=w358:bool, "进站OK"=w357:bool)
        n149 = And(x=w358, y=w357) -> (x .and. y?=w359:bool)
        n150 = case shown="假" w359 {
          tunnel: w368 -> [w373 w385]
          tunnel: [w373 w384] -> w367
          tunnel: w366 -> [w374 w383]
          tunnel: w365 -> [_ w382]
          tunnel: [w374 w381] -> w363
          tunnel: FALSE ("正在运行") -> [w375 w380]
          tunnel: [w375 w379] -> w361
          tunnel: w358 -> [w372 _]
          tunnel: w357 -> [w371 _]
          frame False {
            n151 = case shown="真" w372 {
              tunnel: w371 -> [_ w377]
              frame False {
                n152 = One Button Dialog(message="用户未登录" ("消息")) -> ()  [unwired: 1 in, 1 out]
              }
              frame True {
                n153 = case shown="真" w377 {
                  frame False {
                  }
                  frame True {
                    n154 = One Button Dialog(message="进站失败。" ("消息")) -> ()  [unwired: 1 in, 1 out]
                  }
                }
              }
            }
          }
          frame True {
            n155 = case shown="假" w380 {
              selector: w380 -> [_ w405]
              tunnel: w385 -> [w391 w406]
              tunnel: [w390 w406] -> w384
              tunnel: w383 -> [w389 w407]
              tunnel: w382 -> [w388 _]
              tunnel: [w387 w407] -> w381
              tunnel: [w386 w405] -> w379
              frame False {
                n156 = case shown="真" w389 {
                  tunnel: w391 -> [w392 w397]
                  tunnel: [w392 w396] -> w390
                  tunnel: w388 -> [_ w395]
                  tunnel: [_ w394] -> w387
                  tunnel: [_ TRUE] -> w386
                  frame False {
                  }
                  frame True {
                    n157 = stacked-sequence {
                      tunnel: w397 -> [_ w403 _]
                      tunnel: [_ w402 _] -> w396
                      tunnel: w395 -> [_ w401 _]
                      tunnel: [_ w400 _] -> w394
                      frame #0 {
                        n158 = local write "阻断通讯"(TRUE ("阻断通讯")) -> ()
                      }
                      frame #1 {
                        w399 = cluster{"地址":u16, "布尔":bool, "名称":string}[] [{"地址"=50, "布尔"=TRUE, "名称"="启动"}, {"地址"=51, "布尔"=FALSE, "名称"="停止"}]  # A写入线圈信息组
                        n159 = call "写入单个线圈.vi"("error in"=w403, "写入线圈信息组"=w399, "MB_实体"=w401) -> ("输出簇"=w402:errorcluster, "连接成功"=w400:bool)  [unwired: 7 in]
                      }
                      frame #2 {
                        n160 = local write "阻断通讯"(FALSE ("阻断通讯")) -> ()
                      }
                    }
                  }
                }
              }
              frame True {
              }
            }
          }
        }
        n161 = Bundle By Name(cluster=w364, "正在运行"=w361, "连接成功"=w363) -> (w362:T5)
        n162 = call <vilib>:"Add State(s) to Queue__JKI_lib_State_Machine.vi"("State(s) in (\"\")"=w370) -> ("States Out"=w369:string)  [unwired: 14 in]
      }
      frame "Communication: 设备停止" {
        # "Your code here.\n(You can make a copy of, or modify, this frame)"
        n163 = Unbundle By Name(w413) -> ("serial master instance"=w414:refnum<class "Modbus Master.lvclass">, "连接成功"=w415:bool, "用户登录"=w409:bool)
        n164 = case shown="真" w409 {
          tunnel: w417 -> [w422 w430]
          tunnel: [w422 w429] -> w416
          tunnel: w415 -> [w420 w428]
          tunnel: w414 -> [_ w427]
          tunnel: [w420 w426] -> w412
          tunnel: TRUE ("正在运行") -> [w421 w425]
          tunnel: [w421 w424] -> w410
          frame False {
            n165 = One Button Dialog(message="用户未登录" ("消息")) -> ()  [unwired: 1 in, 1 out]
          }
          frame True {
            n166 = case shown="真" w425 {
              selector: w425 -> [w431 _]
              tunnel: w430 -> [w432 w439]
              tunnel: [w432 w438] -> w429
              tunnel: w428 -> [w433 w437]
              tunnel: w427 -> [_ w436]
              tunnel: [w433 w435] -> w426
              tunnel: [w431 w434] -> w424
              frame False {
              }
              frame True {
                n167 = case shown="真" w437 {
                  tunnel: w439 -> [w441 w446]
                  tunnel: [w441 w445] -> w438
                  tunnel: w436 -> [_ w444]
                  tunnel: [_ w443] -> w435
                  tunnel: [FALSE FALSE] -> w434
                  frame False {
                  }
                  frame True {
                    n168 = stacked-sequence {
                      tunnel: w446 -> [_ w452 _]
                      tunnel: [_ w451 _] -> w445
                      tunnel: w444 -> [_ w450 _]
                      tunnel: [_ w449 _] -> w443
                      frame #0 {
                        n169 = local write "阻断通讯"(TRUE ("阻断通讯")) -> ()
                      }
                      frame #1 {
                        w448 = cluster{"地址":u16, "布尔":bool, "名称":string}[] [{"地址"=50, "布尔"=FALSE, "名称"="启动"}, {"地址"=51, "布尔"=TRUE, "名称"="停止"}]  # A写入线圈信息组
                        n170 = call "写入单个线圈.vi"("error in"=w452, "写入线圈信息组"=w448, "MB_实体"=w450) -> ("输出簇"=w451:errorcluster, "连接成功"=w449:bool)  [unwired: 7 in]
                      }
                      frame #2 {
                        n171 = local write "阻断通讯"(FALSE ("阻断通讯")) -> ()
                      }
                    }
                  }
                }
              }
            }
          }
        }
        n172 = Bundle By Name(cluster=w413, "正在运行"=w410, "连接成功"=w412) -> (w411:T5)
        n173 = call <vilib>:"Add State(s) to Queue__JKI_lib_State_Machine.vi"("State(s) in (\"\")"=w419) -> ("States Out"=w418:string)  [unwired: 14 in]
      }
      frame "Communication: 读运行标志" {
        n174 = Unbundle By Name(w455) -> ("serial master instance"=w454:refnum<class "Modbus Master.lvclass">)
        n175 = stacked-sequence {
          tunnel: w460 -> [_ w469 _]
          tunnel: [_ w468 _] -> w459
          tunnel: [_ w467 _] -> w458
          tunnel: [_ w466 _] -> w457
          tunnel: w454 -> [_ w464 _]
          frame #0 {
            n176 = local write "阻断通讯"(TRUE ("阻断通讯")) -> ()
          }
          frame #1 {
            w465 = T8 [{"地址"=507, "数量"=1, "名称"="1测试结束标志", "线圈组"=[]}]  # A读多组线圈信息组
            n177 = call "读线圈组.vi"("error in"=w469, "读多组线圈__输入"=w465, "MB_实体"=w464) -> ("输出簇"=w468:errorcluster, "正在运行"=w466:bool, "连接成功"=w467:bool)  [unwired: 6 in]
          }
          frame #2 {
            n178 = local write "阻断通讯"(FALSE ("阻断通讯")) -> ()
          }
        }
        n179 = Bundle By Name(cluster=w455, "连接成功"=w458, "正在运行"=w457) -> (w456:T5)
        n180 = call <vilib>:"Add State(s) to Queue__JKI_lib_State_Machine.vi"("State(s) in (\"\")"=w462) -> ("States Out"=w461:string)  [unwired: 14 in]
      }
    }
  }
